vi "Nonlinear Calibration Test.vi"() -> ()   [LabVIEW 2009]
doc: "This example illustrates the use of a calibration grid to calibrate and correct an image for nonlinear distortion and accurate shape measurements.\n\nThis example loads the image of a calibration grid used to calibrate the system, learns the grid, then loads an image of parts acquired using the same setup. The example then corrects the image in two ways. The first method corrects the entire image and then measures the area of the coins. The second method corrects only the area of the coins and displays the difference in processing time."
uses:
  <vilib>/userDefined/High Color/IMAQdx.ctl
  <vilib>/vision/NI_Vision_Development_Module.lvlib
  <vilib>/vision/driver/NI_Vision_Acquisition_Software.lvlib
  Program Files/National Instruments/LabVIEW 2009/resource/objmgr/imaqdx.rc
panel:
  out "Bottom Image 2":T1(plugin-control) caption="Calibrated Measurements"
  out "Top Image 2":T1(plugin-control) caption="Corrected Image"
  in  "Camera Name":T2
  in  "Video Modes":i32(listbox)
  in  "stop":bool
  out "Image":T1(plugin-control)
  out "Buffer Number":u32
  out "Frame Rate":dbl(knob) scale=0.0..100.0 scale format="%.1f"
  in  "Red Range":cluster{"Lower value":i32, "Upper value":i32}={"Lower value"=240, "Upper value"=255}
  in  "Green Range":cluster{"Lower value":i32, "Upper value":i32}={"Lower value"=250, "Upper value"=255}
  in  "Blue Range":cluster{"Lower value":i32, "Upper value":i32}={"Lower value"=250, "Upper value"=255}
  in  "Color Mode":u16(ring) items=["RGB", "HSL", "HSV", "HSI"]
  out "Super Filter":T1(plugin-control)
  out "Bottom Image":T1(plugin-control) caption="Coins Image"
  out "Top Image":T1(plugin-control) caption="Calibration Template"
  # "1. Loads the image of a calibration grid that is used to calibrate the system."
  # "2. Learn the calibration grid. Note that this process is computation intensive and needs a fair amount of time to complete."
  # "3. Load Image of Parts acquired using the same setup."
  # "4. Correct the image and measure areas of the objects in the image."
  # "This step takes measurements in two ways.  The first calculation corrects \nthe entire image, and then takes the measurements.  The second calculation only corrects the coins, and then takes the measurements."
  # "time (ms) to correct entire image, threshold and calculate measurements"
  # "time (ms) to threshold, correct just coins, and then take measurements"
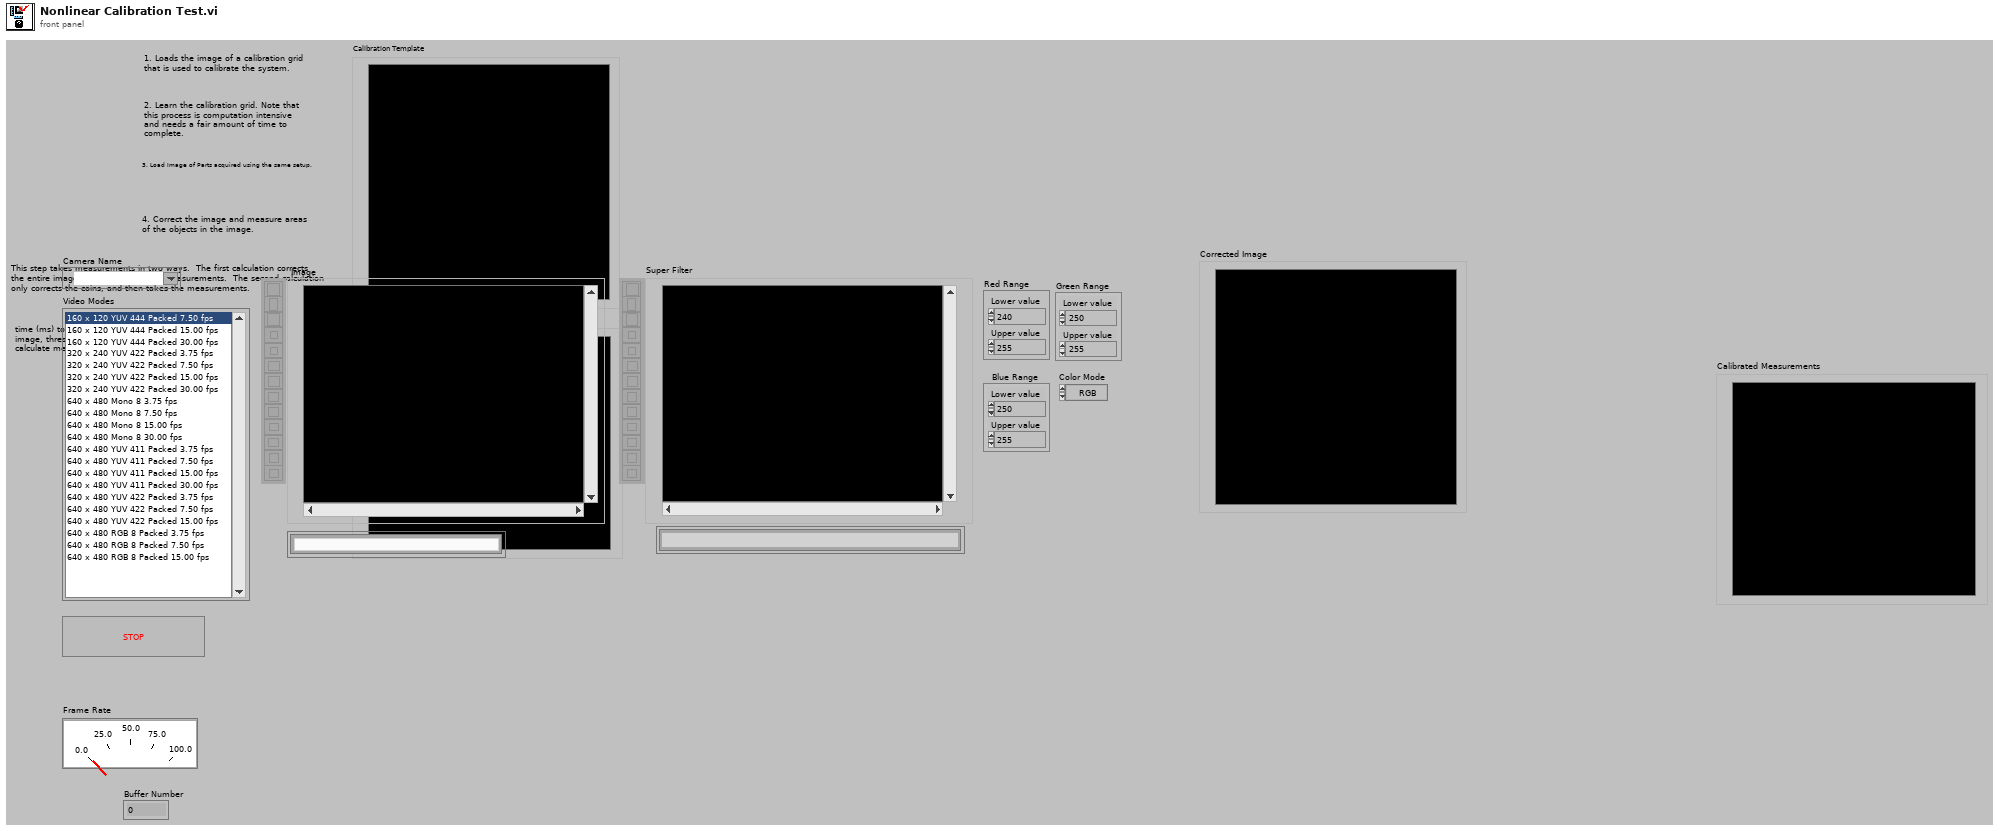
[diagram p1: front panel]
types:
  T1 = typedef "IMAQ Image.ctl" = refnum<image>
  T2 = typedef "IMAQdx.ctl" = refnum<k21>
  T3 = cluster{"X Step":sgl, "Y Step":sgl, "Unit":u32, "Threshold Range":cluster{"Lower value":sgl, "Upper value":sgl}}
  T4 = cluster{"Distortion":u32, "Corrected Image Scaling":u32, "Corrected Image Learn ROI":u32, "Learn Error Map?":bool, "Learn Correction Table?":bool}
  T5 = typedef "Image Type" = u32
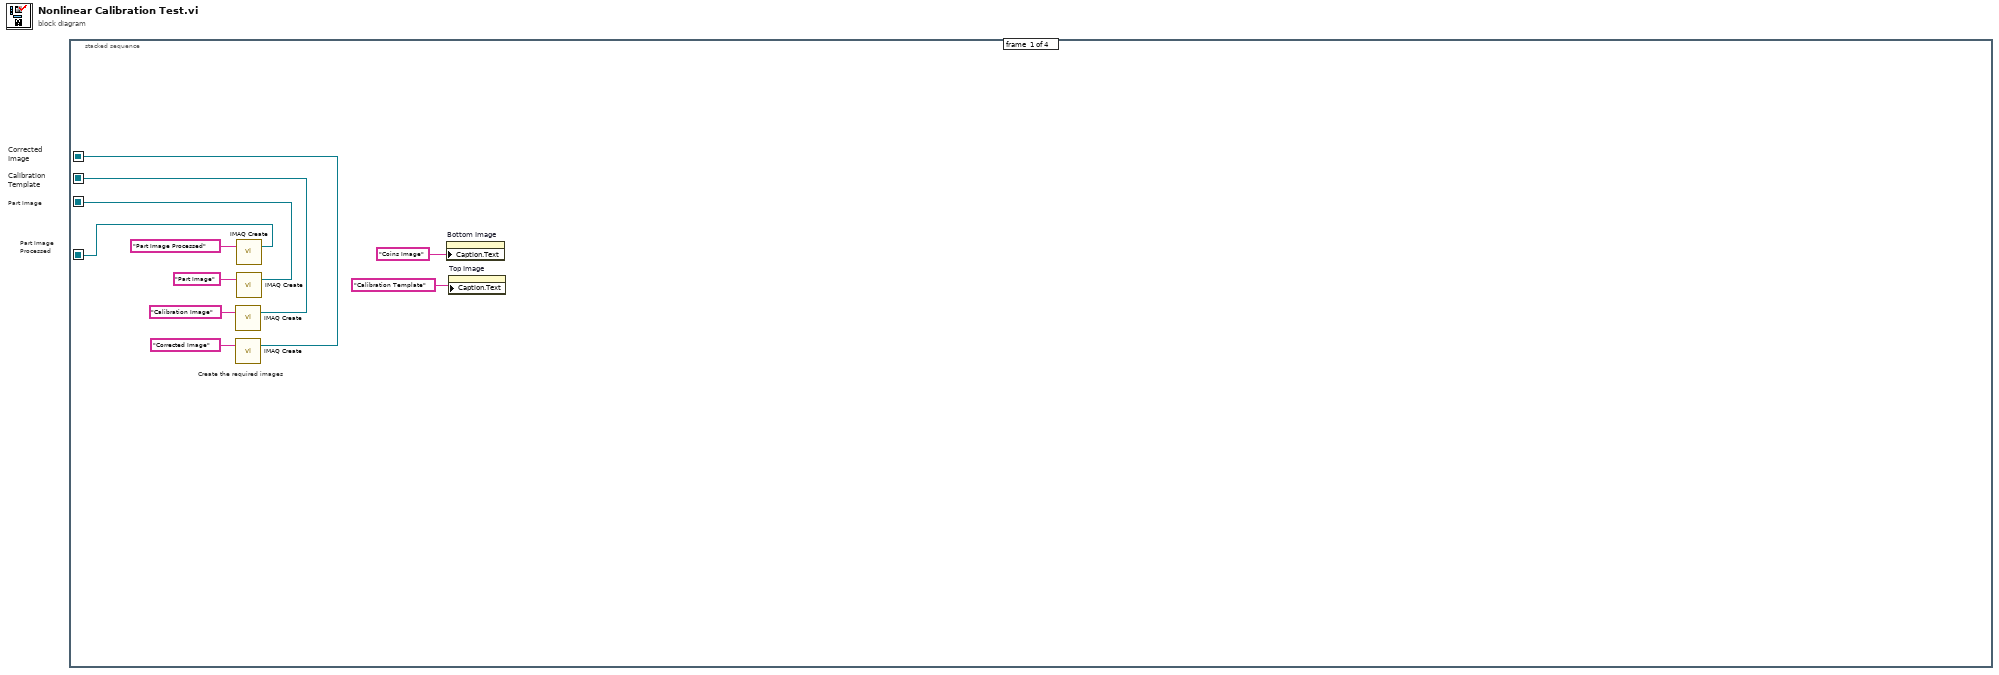
[diagram p0: block diagram]
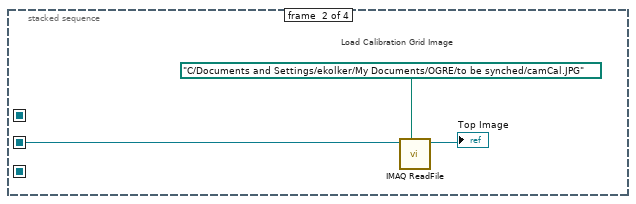
[diagram p2: hidden frame]
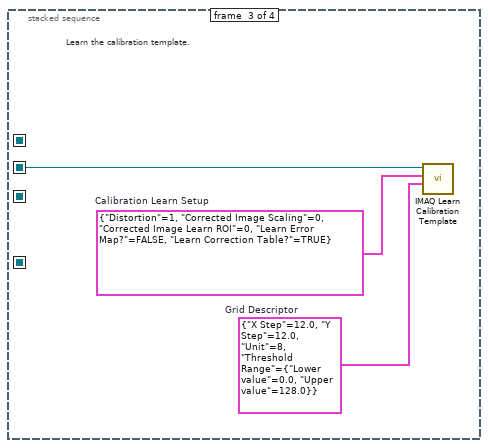
[diagram p3: hidden frame]
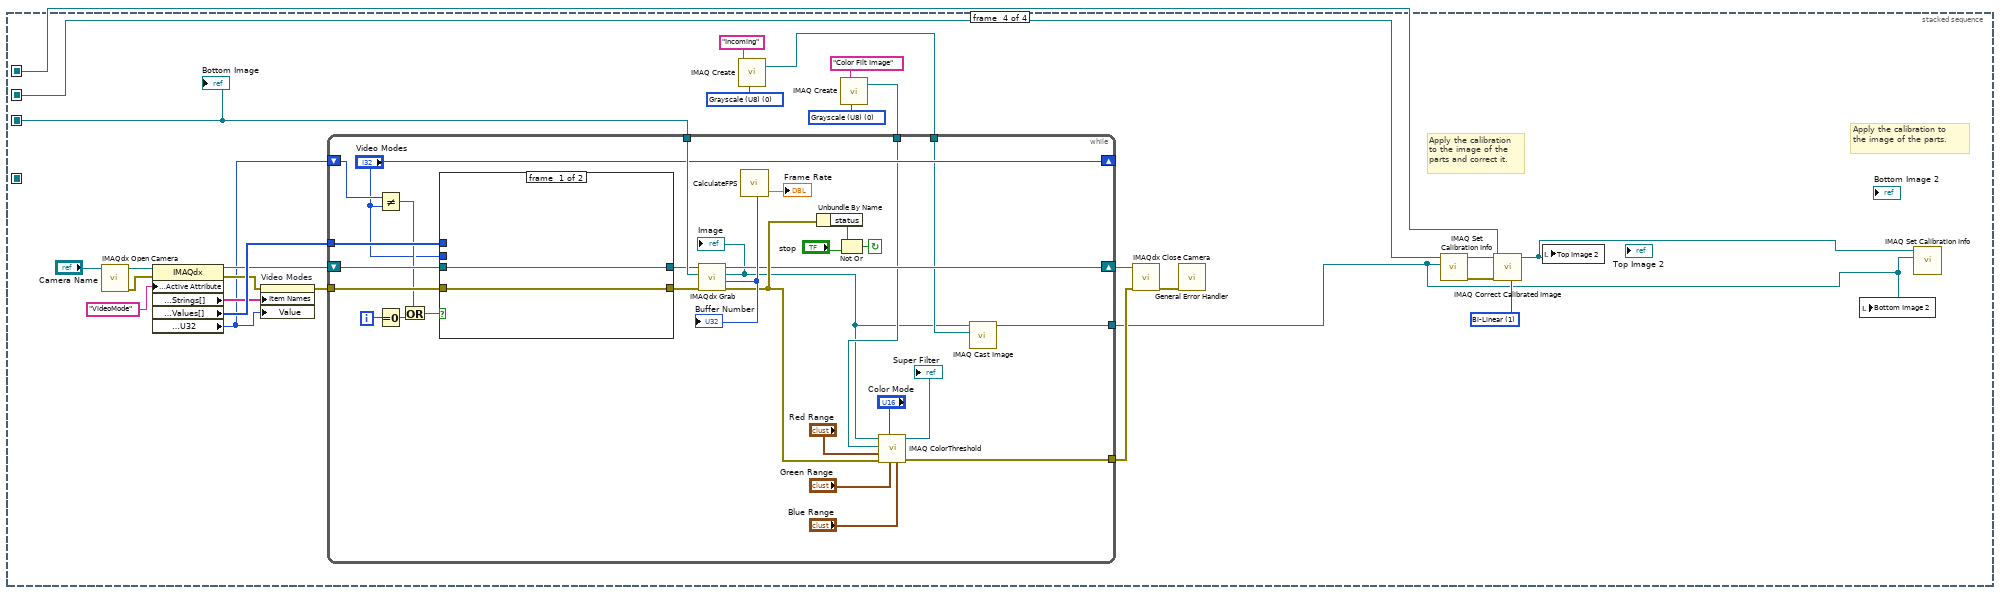
[diagram p4: hidden frame]
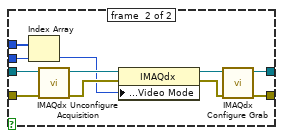
[diagram p5: hidden frame]
diagram:
  # "Corrected\nImage"
  # "Part Image Processed"
  # "Calibration Template"
  # "Part Image"
  n1 = stacked-sequence {
    seq-local: [w9 _ _ _] -> [_ _ _ w19]
    seq-local: [w7 _ _ _] -> [_ w13 w16 w20]
    seq-local: [w5 _ _ _] -> [_ _ _ _]
    seq-local: [w3 _ _ _] -> [_ _ _ w21]
    frame #0 {
      # "Create the required images"
      n2 = call "IMAQ Create"("Image Name"="Calibration Image") -> ("New Image"=w7:T1)  [unwired: 3 in, 2 out]
      n3 = call "IMAQ Create"("Image Name"="Corrected Image") -> ("New Image"=w3:T1)  [unwired: 3 in, 2 out]
      n4 = call "IMAQ Create"("Image Name"="Part Image Processed") -> ("New Image"=w5:T1)  [unwired: 3 in, 2 out]
      n5 = call "IMAQ Create"("Image Name"="Part Image") -> ("New Image"=w9:T1)  [unwired: 3 in, 2 out]
      n6 = property on="Bottom Image" class="ImageControl"("Caption.Text"="Coins Image" ("Title")) -> ()  [unwired: 2 in, 2 out]
      n7 = property on="Top Image" class="ImageControl"("Caption.Text"="Calibration Template" ("Title")) -> ()  [unwired: 2 in, 2 out]
    }
    frame #1 {
      # "Load Calibration Grid Image"
      n8 = call "IMAQ ReadFile"("File Path"=path "C:/Documents and Settings/ekolker/My Documents/OGRE/to be synched/camCal.JPG" ("Calibration Image"), "Image"=w13) -> ("Image Out"=→"Top Image":T1)  [unwired: 3 in, 6 out]
    }
    frame #2 {
      w14 = T3 {"X Step"=12.0, "Y Step"=12.0, "Unit"=8, "Threshold Range"={"Lower value"=0.0, "Upper value"=128.0}}  # Grid Descriptor
      w15 = T4 {"Distortion"=1, "Corrected Image Scaling"=0, "Corrected Image Learn ROI"=0, "Learn Error Map?"=FALSE, "Learn Correction Table?"=TRUE}  # Calibration Learn Setup
      # "Learn the calibration template."
      n9 = call "IMAQ Learn Calibration Template"("Grid Descriptor"=w14, "Calibration Learn Setup"=w15, "Image"=w16) -> ()  [unwired: 4 in, 5 out]
    }
    frame #3 {
      w24 = u32 1 items=["Zero Order", "Bi-Linear", "Quadratic", "Cubic Spline"] ("Interpolation Type")
      w26 = T5 0 items=["Grayscale (U8)", "Grayscale (I16)", "Grayscale (SGL)", "Complex (CSG)", "RGB (U32)", "HSL (U32)", "RGB (U64)", "Grayscale (U16)"] ("Image Type")
      w29 = T5 0 items=["Grayscale (U8)", "Grayscale (I16)", "Grayscale (SGL)", "Complex (CSG)", "RGB (U32)", "HSL (U32)", "RGB (U64)", "Grayscale (U16)"] ("Image Type")
      # "Apply the calibration to the image of the parts."
      # "Apply the calibration to the image of the parts and correct it."
      n10 = call <vilib>:"IMAQdx Open Camera.vi"("Session In"="Camera Name") -> ("error out"=w38:errorcluster, "Session Out"=w41:T2)  [unwired: 2 in, 7 out]
      n11 = property class="IMAQdx"(reference=w41, error in=w38, "Camera Attributes:Active Attribute"="VideoMode" ("ActiveAttribute")) -> (reference out=w36:T2, error out=w37:errorcluster, "Camera Attributes:Enum:Strings[]"=w34:string[], "Camera Attributes:Enum:Values[]"=w39:u32[], "Camera Attributes:Value:U32"=w33:u32)
      n12 = property on="Video Modes" class="ListBox (strict)"(error in=w37, "Item Names"=w34, "Value"=w33) -> (error out=w35:errorcluster)  [unwired: 1 in, 1 out]
      n13 = call "IMAQ Create"("Image Name"="Incoming", "Image Type"=w26) -> ("New Image"=w25:T1)  [unwired: 2 in, 2 out]
      n14 = call "IMAQ Create"("Image Name"="Color Filt Image", "Image Type"=w29) -> ("New Image"=w30:T1)  [unwired: 2 in, 2 out]
      n15 = while {
        tunnel: w39 -> [w69]
        shift-left: w33 -> [w57]
        shift-right: ["Video Modes"] -> _
        tunnel: w19 -> [w70]
        tunnel: w35 -> [w71]
        shift-right: [w50] -> w43
        shift-left: w36 -> [w72]
        tunnel: w30 -> [w49]
        tunnel: [w48] -> w28
        tunnel: w25 -> [w46]
        tunnel: [w44] -> w17
        i -> [w63]
        stop <- w66 continue-if-true
        n16 = Not Equal?(x=w57, y="Video Modes") -> (x != y?=w64:bool)
        n17 = Equal To 0?(x=w63) -> (x = 0?=w62:bool)
        n18 = Or(x=w64, y=w62) -> (x .or. y?=w65:bool)
        n19 = case shown="True" w65 {
          tunnel: w72 -> [w74 w83]
          tunnel: w71 -> [w73 w82]
          tunnel: [w74 w79] -> w60
          tunnel: [w73 w80] -> w61
          tunnel: w69 -> [_ w85]
          tunnel: "Video Modes" -> [_ w84]
          frame #0 {
          }
          frame #1 {
            n20 = Index Array(array=w85, index=w84) -> (element=w75:u32)
            n21 = call <vilib>:"IMAQdx Unconfigure Acquisition.vi"("error in"=w82, "Session In"=w83) -> ("error out"=w76:errorcluster, "Session Out"=w81:T2)  [unwired: 8 out]
            n22 = property class="IMAQdx"(reference=w81, error in=w76, "Acquisition Attributes:Video Mode"=w75) -> (reference out=w78:T2, error out=w77:errorcluster)
            n23 = call <vilib>:"IMAQdx Configure Grab.vi"("error in"=w77, "Session In"=w78) -> ("error out"=w80:errorcluster, "Session Out"=w79:T2)  [unwired: 1 in, 7 out]
          }
        }
        n24 = call <vilib>:"IMAQdx Grab.vi"("error in"=w61, "Image In"=w70, "Session In"=w60) -> ("error out"=w55:errorcluster, "Buffer Number Out"=w58:u32, "Image Out"=w45:T1, "Session Out"=w50:T2)  [unwired: 1 in, 4 out]
        "Image" <- w45
        "Buffer Number" <- w58
        n25 = call "CalculateFPS.vi"("buffer number"=w58) -> ("processed FPS"=→"Frame Rate":dbl)  [unwired: 2 out]
        n26 = Unbundle By Name(w55) -> ("status"=w67:bool)
        n27 = Not Or(1:"stop", 2:w67) -> (0:w66:bool)
        n28 = call "IMAQ ColorThreshold"("Blue or Luma or Val or Inten Range"="Blue Range", "Green or Sat Range"="Green Range", "Color Mode"="Color Mode", "error in (no error)"=w55, "Red or Hue Range"="Red Range", "Image Dst"=w49, "Image Src"=w45) -> ("error out"=w48:errorcluster, "Image Dst Out"=→"Super Filter":T1)  [unwired: 3 in]
        n29 = call "IMAQ Cast Image"("Image Dst"=w46, "Image Src"=w45) -> ("Image Dst Out"=w44:T1)  [unwired: 8 in, 1 out]
      }
      n30 = call <vilib>:"IMAQdx Close Camera.vi"("error in"=w28, "Session In"=w43) -> ("error out"=w32:errorcluster)  [unwired: 9 out]
      n31 = call <vilib>:"General Error Handler.vi"("error in (no error)"=w32) -> ()  [unwired: 1 in, 14 out]
      n32 = call "IMAQ Set Calibration Info"("Image Dst"=w17, "Image Src"=w20) -> ("error out"=w22:errorcluster, "Calibrated Image"=w23:T1)  [unwired: 2 in, 6 out]
      n33 = call "IMAQ Correct Calibrated Image"("Interpolation Type"=w24, "error in (no error)"=w22, "Image Dst"=w21, "Image Src"=w23) -> ("Corrected Image"=w18:T1)  [unwired: 3 in, 4 out]
      n34 = local write "Top Image 2"(w18) -> ()
      n35 = local write "Bottom Image 2"(w17) -> ()
      n36 = call "IMAQ Set Calibration Info"("Image Dst"=w17, "Image Src"=w18) -> ()  [unwired: 2 in, 8 out]
      "Bottom Image" <- w19
    }
  }
